vi "clipcomprobation.vi"(0 "input cluster":T1, 1 "Channels values 2":i32[](array[numeric]), 2 "vclip":i32[](array[numeric]), 5 "Channels init":i32[](array[numeric])=[2000], 7 "Boolean":bool, 11 "error out 2":errorcluster, 12 "Number points":i32) -> (4 "L1  values":i32[](array[numeric]), 6 "XY Graph":cluster{"Y":dbl[], "Y":dbl[]}[](graph), 10 "XY Graph 2":cluster{"Y":dbl[], "Y":dbl[]}[](graph), 15 "error out":errorcluster)   [LabVIEW 2009]
uses:
  <vilib>/Utility/NIReport.llb/NI_report.lvclass
  <vilib>/Analysis/NI_AALPro.lvlib
panel:
  in  "Array":dbl[](array[numeric])=[0.05, 0.1, 0.2, 0.3, 0.4, 0.5, 0.6, 0.7, 0.8, 0.9, 1.0, 1.2, 1.4, 1.6, 1.8, 2.0, 2.2, 2.5]
  in  "L1  50% invented":dbl[][](array[numeric])
  in  "L1 min invented":i32[](array[numeric])=[242, 504, 1031, 2128, 3263, 4418, 5634, 6888]
  out "L1  50%":dbl[][](array[numeric])=[[182.05332645693656, 181.0458957661739, 182.31328051706822, 182.44384615384615, 179.9591580860661, 183.67138786049767, 183.0415079653926], [383.1443079334591, 380.3408546343534, 383.09068068207546, 382.9081242164992, 377.8888565224893, 386.4745006061593, 384.33733278296165], [789.794916143154, 783.9334435523022, 789.880331635444, 788.1638578058222, 779.1397265900023, 796.380113600458, 792.3805482207972], [1637.2849189817332, 1624.3008579976345, 1635.9791868307739, 1633.4037928039274, 1613.351662874732, 1647.9524154468106, 1640.5214046384517], [2513.43820756283, 2496.681867952526, 2512.120672224883, 2508.5174246445135, 2478.2432072662637, 2532.0838659445626, 2519.7319162836616], [4350.429616233692, 4325.797863663112, 4346.430175185175, 4343.835753463216, 4286.1263991243895, 4381.02010040906, 4360.577157137679], [5321.96395522116, 5291.780098348377, 5317.9835218197695, 5305.673007498198, 5228.362955923682, 5348.7398745375585, 5316.2612416656], [6878.716199794284, 6844.2297782699125, 6886.512941570447, 6849.728580417201, 6743.132495285984, 6910.301756503628, 6900.4988799604525]]
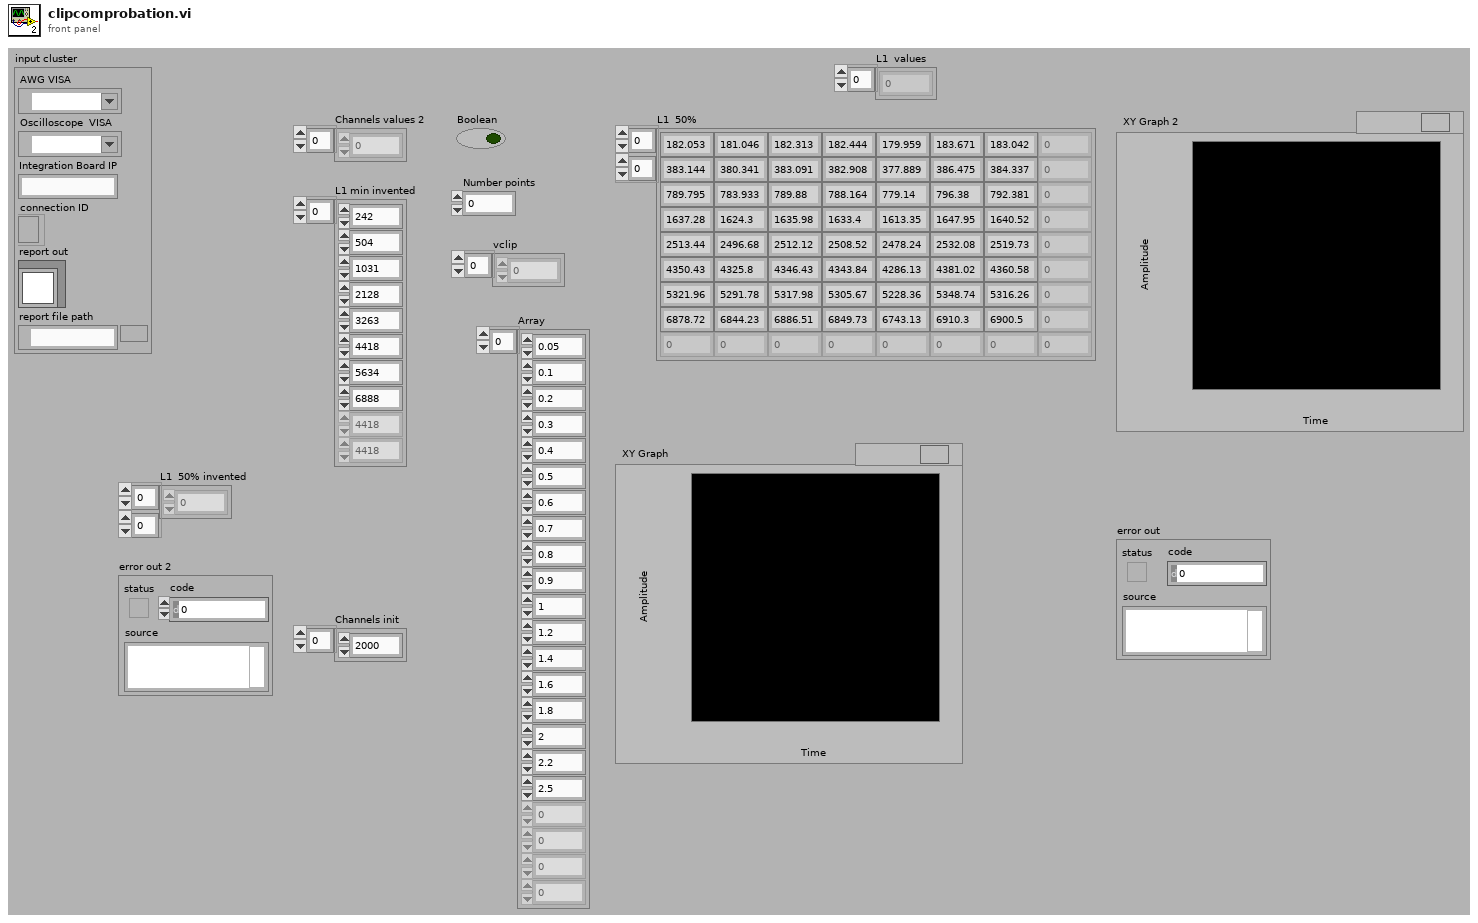
[diagram p1: front panel]
types:
  T1 = cluster{"AWG VISA":refnum<visa-resource-name>, "Oscilloscope  VISA ":refnum<visa-resource-name>, "Integration Board IP":string, "connection ID":refnum<k5>, "report out":refnum<class "NI_report.lvclass">, "report file path":path}
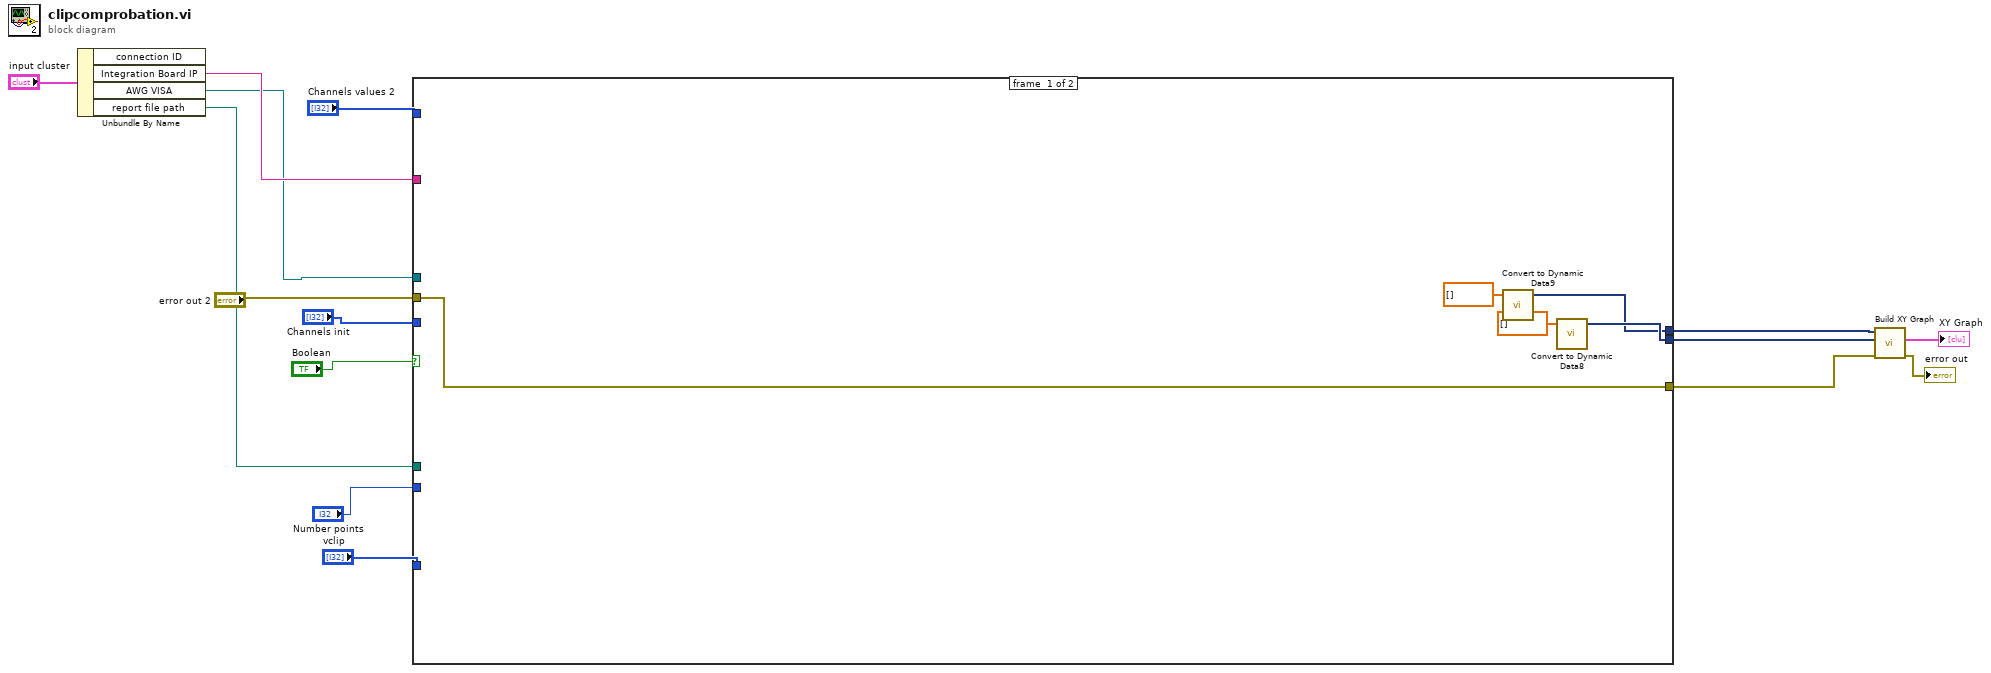
[diagram p0: block diagram]
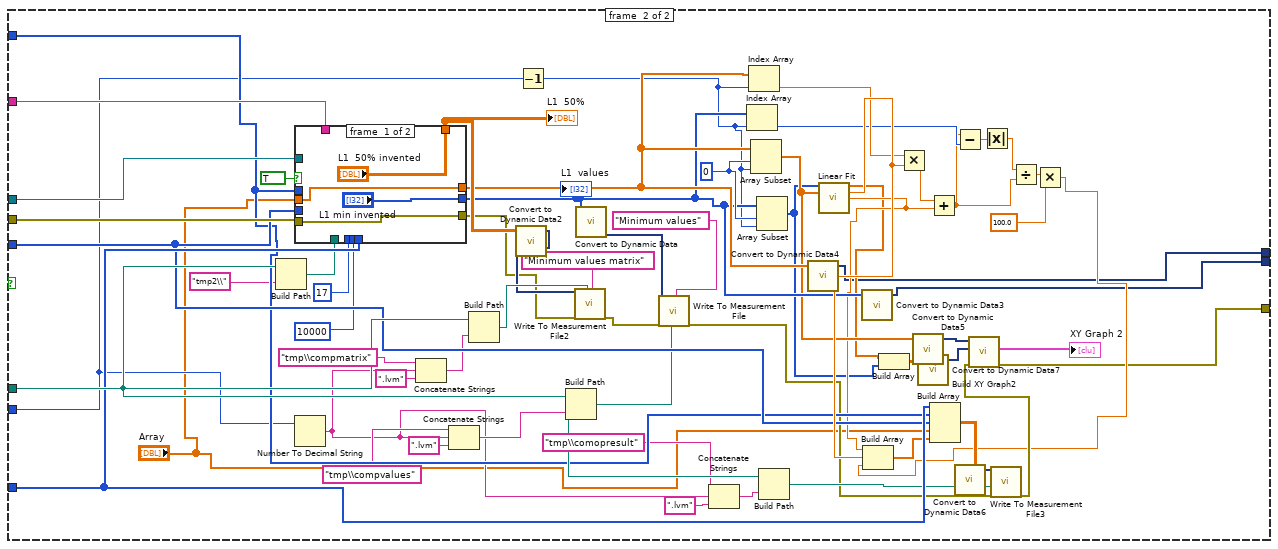
[diagram p2: hidden frame]
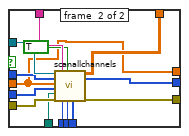
[diagram p3: hidden frame]
diagram:
  n1 = Unbundle By Name("input cluster") -> ("Integration Board IP"=w10:string, "AWG VISA"=w9:refnum<visa-resource-name>, "report file path"=w8:path)  [unwired: 1 out]
  n2 = case shown="True" "Boolean" {
    tunnel: "error out 2" -> [w20 w84]
    tunnel: w9 -> [_ w83]
    tunnel: w10 -> [_ w82]
    tunnel: w8 -> [_ w81]
    tunnel: "vclip" -> [_ w79]
    tunnel: "Channels init" -> [_ w78]
    tunnel: "Channels values 2" -> [_ w77]
    tunnel: [w20 w24] -> w4
    tunnel: "Number points" -> [_ w76]
    tunnel: [w19 w23] -> w2
    tunnel: [w18 w22] -> w1
    frame #0 {
      n3 = call "Convert to Dynamic Data9"("Array"=dbl[] []) -> ("Dynamic Data Type"=w18:dynamicdata)  [unwired: 3 in]
      n4 = call "Convert to Dynamic Data8"("Array"=dbl[] []) -> ("Dynamic Data Type"=w19:dynamicdata)  [unwired: 3 in]
    }
    frame #1 {
      w63 = 0 ("length")
      n5 = Build Path(base path=w81, name or relative path="tmp2\\") -> (appended path=w71:path)
      n6 = case shown="True" TRUE {
        tunnel: [w88 w102] -> w65
        tunnel: w84 -> [w88 w101]
        tunnel: w83 -> [_ w100]
        tunnel: w82 -> [_ w99]
        tunnel: w78 -> [_ w98]
        tunnel: "Array" -> [w85 w89]
        tunnel: w77 -> [_ w97]
        tunnel: 17 ("Value") -> [_ w96]
        tunnel: 10000 ("Value") -> [_ w95]
        tunnel: ["L1 min invented" w93] -> w52
        tunnel: w71 -> [_ w92]
        tunnel: w79 -> [_ w91]
        tunnel: ["L1  50% invented" w90] -> w67
        tunnel: [w85 w89] -> w55
        frame #0 {
        }
        frame #1 {
          n7 = call "scanallchannels.vi"("VISA resource name out"=w100, "nm ch"=w97, "Voltages values"=w89, "Init ch value"=w98, "base path"=w92, "error in"=w101, "Integration Board IP"=w99, "L1 Address"=w96, "Save test data"=TRUE, "Ch burst"=w95, "vclip"=w91) -> ("L1  50%"=w90:dbl[][], "L1 min values"=w93:i32[], "error out"=w102:errorcluster)  [unwired: 6 in]
        }
      }
      "L1  50%" <- w67
      "L1  values" <- w52
      n8 = Number To Decimal String(number=w76) -> (decimal integer string=w30:string)  [unwired: 1 in]
      n9 = Concatenate Strings("tmp\\compmatrix" ("name or relative path"), w30, ".lvm" ("string")) -> (w32:string)
      n10 = Concatenate Strings("tmp\\compvalues" ("name or relative path"), w30, ".lvm" ("string")) -> (w33:string)
      n11 = Build Path(base path=w81, name or relative path=w32) -> (appended path=w68:path)
      n12 = call "Convert to Dynamic Data2"("2D Array"=w67) -> ("Dynamic Data Type"=w66:dynamicdata)  [unwired: 3 in]
      n13 = Decrement(x=w76) -> (x-1=w38:i32)
      n14 = Build Path(base path=w81, name or relative path=w33) -> (appended path=w73:path)
      n15 = call "Write To Measurement File2"("Signals"=w66, "error in (no error)"=w65, "Filename"=w68, "Comment"="Minimum values matrix") -> ("error out"=w64:errorcluster)  [unwired: 13 in, 2 out]
      n16 = call "Convert to Dynamic Data"("Array"=w52) -> ("Dynamic Data Type"=w75:dynamicdata)  [unwired: 3 in]
      n17 = call "Write To Measurement File"("Signals"=w75, "error in (no error)"=w64, "Filename"=w73, "Comment"="Minimum values") -> ("error out"=w48:errorcluster)  [unwired: 13 in, 2 out]
      n18 = Concatenate Strings("tmp\\comopresult" ("name or relative path"), w30, ".lvm" ("string")) -> (w28:string)
      n19 = Index Array(array=w52, index=w38) -> (element=w56:i32)
      n20 = Index Array(array=w55, index=w38) -> (element=w62:dbl)
      n21 = Array Subset(array=w55, index=w63, length=w38) -> (w51:dbl[])
      n22 = Array Subset(array=w52, index=w63, length=w38) -> (w41:i32[])
      n23 = Build Path(base path=w81, name or relative path=w28) -> (appended path=w49:path)
      n24 = call "Convert to Dynamic Data4"("Array"=w55) -> ("Dynamic Data Type"=w22:dynamicdata)  [unwired: 3 in]
      n25 = call <vilib>:"Linear Fit.vi"("Y"=w41, "X"=w51) -> ("Best Linear Fit"=w42:dbl[], "slope"=w80:dbl, "intercept"=w47:dbl)  [unwired: 9 in, 2 out]
      n26 = call "Convert to Dynamic Data3"("Array"=w52) -> ("Dynamic Data Type"=w23:dynamicdata)  [unwired: 3 in]
      n27 = Build Array(w42, w41) -> (w40:dbl[][])
      n28 = Multiply(x=w62, y=w80) -> (x*y=w61:dbl)
      n29 = call "Convert to Dynamic Data5"("Array"=w51) -> ("Dynamic Data Type"=w54:dynamicdata)  [unwired: 3 in]
      n30 = call "Convert to Dynamic Data7"("2D Array"=w40) -> ("Dynamic Data Type"=w39:dynamicdata)  [unwired: 3 in]
      n31 = Add(x=w61, y=w47) -> (x+y=w50:dbl)
      n32 = Subtract(x=w50, y=w56) -> (x-y=w60:dbl)
      n33 = Absolute Value(x=w60) -> (abs(x)=w59:dbl)
      n34 = Divide(x=w59, y=w50) -> (x/y=w58:dbl)
      n35 = Multiply(x=w58, y=100.0) -> (x*y=w25:dbl)
      n36 = Build Array(w47, w80, w25) -> (w46:dbl[])
      n37 = Build Array(w79, w77, w78, "Array", w46) -> (w45:dbl[][])
      n38 = call "Convert to Dynamic Data6"("2D Array"=w45) -> ("Dynamic Data Type"=w44:dynamicdata)  [unwired: 3 in]
      n39 = call "Write To Measurement File3"("Signals"=w44, "error in (no error)"=w48, "Filename"=w49) -> ("error out"=w43:errorcluster)  [unwired: 14 in, 2 out]
      n40 = call "Build XY Graph2"("error in (no error)"=w43, "Y Input"=w39, "X Input"=w54) -> ("error out"=w24:errorcluster, "XY Graph"=→"XY Graph 2":cluster{"Y":dbl[], "Y":dbl[]}[])  [unwired: 7 in]
    }
  }
  n41 = call "Build XY Graph"("error in (no error)"=w4, "Y Input"=w2, "X Input"=w1) -> ("error out"=→"error out":errorcluster, "XY Graph"=→"XY Graph":cluster{"Y":dbl[], "Y":dbl[]}[])  [unwired: 7 in]
